vi "HOST_feedback+datatrig_AAoptAOD_9-11-23.vi"() -> ()   [LabVIEW 2020]
uses:
  <vilib>/rvi/interface/nirviMethod/nirviMethod.xnode
  <vilib>/rvi/errors/niLvFpgaMergeErrorWithErrorCode.vi
  <instrlib>/_niInstr/Streaming/v1/Host/niInstr Streaming v1 Host.lvlib
  <vilib>/rvi/interface/nirviReadWriteControl/nirviReadWriteControl.xnode
  <vilib>/rvi/interface/nirviCloseFPGA/nirviCloseFPGA.xnode
  <vilib>/rvi/interface/nirviOpenFPGA/nirviOpenFPGA.xnode
  <vilib>/rvi/interface/Simulation/niFpgaSimulationCallBeginRW.vi
  <vilib>/rvi/errors/niLvFpgaAdjustHostInterfaceError.vi
  NiFpgaLv.dll
  <vilib>/Utility/error.llb/Error Cluster From Error Code.vi
  <vilib>/Utility/file.llb/Write Delimited Spreadsheet (string).vi
  <instrlib>/_niInstr/Streaming/v1/Host/Public/Start Finite Stream.vi
  <instrlib>/_niInstr/Streaming/v1/Host/Public/Wait for Stream.vi
  <vilib>/FPGAPlugInAG/Dynamic/niLvFpga_ConfigureFifo_Dynamic.vi
  <vilib>/FPGAPlugInAG/Dynamic/niLvFpga_StartFifo_Dynamic.vi
  <vilib>/FPGAPlugInAG/Dynamic/niLvFpga_ReadFifo_Dynamic.vi
  <vilib>/FPGAPlugInAG/Dynamic/niLvFpga_WriteFifo_Dynamic.vi
  <vilib>/FPGAPlugInAG/Dynamic/niLvFpga_Close_Dynamic.vi
  FPGA Bitfiles/rfsignal_FPGATarget_feedbackarray+da_BHXJFx-D6v4.lvbitx
  <vilib>/measure/NI_MAPro.lvlib
  <instrlib>/_niInstr/Streaming/v1/Host/Public/Start Continuous Stream.vi
  <vilib>/measure/maspectr.llb/FFT Power Spectrum and PSD for N Chan.vi
  <vilib>/FPGAPlugInAG/PXIe-7972R/niLvFpga_Open_PXIe-7972R.vi
  <vilib>/rvi/interface/common/dynamic/niFpgaDynamicAddResources.vi
  <vilib>/userdefined/Silver/nirio_resource_slv.ctl
  Controls/Clock Select.ctl
  PID/Typedef/niFpgaPID_PIDGains.ctl
  PID/Typedef/niFpgaPID_OutputRange.ctl
  PID/Typedef/niFpgaPID_SetpointWeightings.ctl
  PID/Typedef/niFpgaPID_PIDActions.ctl
panel:
  in  "RF Power normalize":bool=TRUE
  in  "Save data":bool
  in  "File name":string="Z_3mbar_i"
  in  "Save Path Directory":path=path "D:/Lab Data/test"
  out "SUM PSD":cluster{"f0":dbl, "df":dbl, "magnitude":dbl[]}[](graph)
  out "SUM":waveform(dbl)[](graph)=[{"t0"=timestamp(0 s since 1904-01-01), "dt"=0.0002, "Y"=array[1000 elements]}, {"t0"=timestamp(0 s since 1904-01-01), "dt"=0.0002, "Y"=array[1000 elements]}, {"t0"=timestamp(0 s since 1904-01-01), "dt"=0.0002, "Y"=array[1000 elements]}, {"t0"=timestamp(0 s since 1904-01-01), "dt"=0.0002, "Y"=array[1000 elements]}]
  out "Y PSD":cluster{"f0":dbl, "df":dbl, "magnitude":dbl[]}[](graph)
  out "Y":waveform(dbl)[](graph)=[{"t0"=timestamp(0 s since 1904-01-01), "dt"=0.0002, "Y"=array[1000 elements]}, {"t0"=timestamp(0 s since 1904-01-01), "dt"=0.0002, "Y"=array[1000 elements]}, {"t0"=timestamp(0 s since 1904-01-01), "dt"=0.0002, "Y"=array[1000 elements]}, {"t0"=timestamp(0 s since 1904-01-01), "dt"=0.0002, "Y"=array[1000 elements]}]
  out "X PSD":cluster{"f0":dbl, "df":dbl, "magnitude":dbl[]}[](graph)
  out "X":waveform(dbl)[](graph)=[{"t0"=timestamp(0 s since 1904-01-01), "dt"=0.0002, "Y"=array[1000 elements]}, {"t0"=timestamp(0 s since 1904-01-01), "dt"=0.0002, "Y"=array[1000 elements]}, {"t0"=timestamp(0 s since 1904-01-01), "dt"=0.0002, "Y"=array[1000 elements]}, {"t0"=timestamp(0 s since 1904-01-01), "dt"=0.0002, "Y"=array[1000 elements]}]
  in  "Set Point Initialization":bool
  in  "Feedback scaling y":fxp<+,25,4>
  in  "Gains Y":T1[](array[typedef]) {"filter coefficient" min=0 max=1; "proportional gain" step=0.125}
  in  "Gains X":T1[](array[typedef]) {"filter coefficient" min=0 max=1; "proportional gain" step=0.125}
  in  "Data transfer method":bool
  in  "Downsample":u16=1
  in  "Signal Delay (us)":i32=5
  out "actions":T2
  out "error":sgl
  out "output":sgl
  out "error 2":sgl
  out "error 3":sgl
  out "output 3":sgl
  out "actions 3":T2
  out "output 2":sgl
  out "actions 2":T2
  in  "Gains Z":T1[](array[typedef]) {"filter coefficient" min=0 max=1; "proportional gain" step=0.125}
  in  "setpoint weighting 3":T3={"proportional weighting (1)"=1.0, "derivative weighting (0)"=0.0} {"derivative weighting (0)" min=0 max=1; "proportional weighting (1)" min=0 max=1}
  in  "output range 3":T4={"output high (Inf)"=inf, "output low (-Inf)"=-inf}
  in  "Z reset? (F)":bool
  in  "setpoint weighting 2":T3={"proportional weighting (1)"=1.0, "derivative weighting (0)"=0.0} {"derivative weighting (0)" min=0 max=1; "proportional weighting (1)" min=0 max=1}
  in  "output range 2":T4={"output high (Inf)"=inf, "output low (-Inf)"=-inf}
  in  "Y reset? (F)":bool
  in  "Feedback scaling z":fxp<+,32,4>
  in  "Feedback scaling x":fxp<+,25,4>
  in  "Apply feedback":bool
  in  "Data Trigger Level (V)":dbl
  in  "Record Size":u32=1024
  out "AI":waveform(dbl)[](graph)
  in  "Data Trigger When":enum8{"Trigger Above", "Trigger Below"}(ring)
  in  "Trigger Type":enum8{"Immediate", "Data Trigger", "TRIG input"}(ring)
  in  "Direction switch":bool
  in  "Step gain values":dbl
  in  "?":bool
  in  "% of max CH 1":dbl=85.0
  in  "% of max CH 0":dbl=90.0
  in  "setpoint weighting":T3={"proportional weighting (1)"=1.0, "derivative weighting (0)"=0.0} {"derivative weighting (0)" min=0 max=1; "proportional weighting (1)" min=0 max=1}
  in  "output range":T4={"output high (Inf)"=inf, "output low (-Inf)"=-inf}
  in  "X reset? (F)":bool
  in  "write time ch0":bool
  in  "Record time for power sweep CH0":bool
  in  "Record time for power sweep CH1":bool
  in  "write time ch1":bool
  in  "save path for power calibration (dialog if empty)":path
  out "time check":u16=16
  in  "Cycles per step":u16=30
  in  "Gain Scan Endpoint (CH1)":dbl[](array[numeric])=[100.0, 100.0, 100.0, 100.0, 100.0, 100.0, 100.0, 100.0, 100.0, 100.0, 100.0, 100.0, 100.0, 100.0, 100.0, 100.0, 100.0, 100.0, 100.0, 100.0, 100.0, 100.0, 100.0, 100.0, 100.0, 100.0, 100.0, 100.0, 100.0, 100.0, 100.0, 100.0, 100.0, 100.0, 100.0, 100.0]
  in  "Gain Scan Endpoint (CH0)":dbl[](array[numeric])=[100.0, 100.0, 100.0, 100.0, 100.0, 100.0, 100.0, 100.0, 100.0, 100.0, 100.0, 100.0, 100.0, 100.0, 100.0, 100.0, 100.0, 100.0, 100.0, 100.0, 100.0, 100.0, 100.0, 100.0, 100.0, 100.0, 100.0, 100.0, 100.0, 100.0, 100.0, 100.0, 100.0, 100.0, 100.0, 100.0]
  in  "Scan End Setpoint (CH1)":dbl[](array[numeric])=[23.0, 24.0, 25.0, 26.0, 27.0, 28.0, 23.0, 24.0, 25.0, 26.0, 27.0, 28.0, 23.0, 24.0, 25.0, 26.0, 27.0, 28.0, 23.0, 24.0, 25.0, 26.0, 27.0, 28.0, 23.0, 24.0, 25.0, 26.0, 27.0, 28.0, 23.0, 24.0, 25.0, 26.0, 27.0, 28.0] format="%#_10f"
  in  "Scan CH1":bool
  in  "Scan CH0":bool
  in  "Fq Scan Endpoint (CH0)":dbl[](array[numeric])=[23.0, 23.0, 23.0, 23.0, 23.0, 23.0, 24.0, 24.0, 24.0, 24.0, 24.0, 24.0, 25.0, 25.0, 25.0, 25.0, 25.0, 25.0, 26.0, 26.0, 26.0, 26.0, 26.0, 26.0, 27.0, 27.0, 27.0, 27.0, 27.0, 27.0, 28.0, 28.0, 28.0, 28.0, 28.0, 28.0] format="%#_10f"
  in  "Gain Scan Step Size % (CH1)":dbl=1.0
  in  "Gain Scan Step Size % (CH0)":dbl=1.0
  in  "Fq Scan Step Size MHz (CH1)":dbl=0.1
  in  "Fq Scan Step Size MHz (CH0)":dbl=0.1
  in  "Input pass through\nmode":enum16{"Wire", "Accum-edge"}(ring)=enum."Accum-edge"
  in  "# of beams":u8=36
  in  "Wave Reader CH 1 (MHz)":dbl[](array[numeric])=[23.0, 24.0, 25.0, 26.0, 27.0, 28.0, 23.0, 24.0, 25.0, 26.0, 27.0, 28.0, 23.0, 24.0, 25.0, 26.0, 27.0, 28.0, 23.0, 24.0, 25.0, 26.0, 27.0, 28.0, 23.0, 24.0, 25.0, 26.0, 27.0, 28.0, 23.0, 24.0, 25.0, 26.0, 27.0, 28.0] format="%#_15f"
  in  "Gain CH 1 (%)":dbl[](array[numeric])=[100.0, 100.0, 100.0, 100.0, 100.0, 100.0, 100.0, 100.0, 100.0, 100.0, 100.0, 100.0, 100.0, 100.0, 100.0, 100.0, 100.0, 100.0, 100.0, 100.0, 100.0, 100.0, 100.0, 100.0, 100.0, 100.0, 100.0, 100.0, 100.0, 100.0, 100.0, 100.0, 100.0, 100.0, 100.0, 100.0]
  in  "Remove transition edges":i32=5
  in  "Time per beam in us":i32=20
  in  "stop":bool
  in  "Gain CH 0 (%)":dbl[](array[numeric])=[100.0, 100.0, 100.0, 100.0, 100.0, 100.0, 100.0, 100.0, 100.0, 100.0, 100.0, 100.0, 100.0, 100.0, 100.0, 100.0, 100.0, 100.0, 100.0, 100.0, 100.0, 100.0, 100.0, 100.0, 100.0, 100.0, 100.0, 100.0, 100.0, 100.0, 100.0, 100.0, 100.0, 100.0, 100.0, 100.0]
  in  "Wave Reader CH 0 (MHz)":dbl[](array[numeric])=[23.0, 23.0, 23.0, 23.0, 23.0, 23.0, 24.0, 24.0, 24.0, 24.0, 24.0, 24.0, 25.0, 25.0, 25.0, 25.0, 25.0, 25.0, 26.0, 26.0, 26.0, 26.0, 26.0, 26.0, 27.0, 27.0, 27.0, 27.0, 27.0, 27.0, 28.0, 28.0, 28.0, 28.0, 28.0, 28.0] format="%#_13f"
  in  "Magnitude Initialization Vpp":dbl[](array[numeric])=[1.0, 1.0] format="%0.2p"
  in  "Frequencies (Hz)":dbl[](array[numeric])=[10000.0, 10000.0] format="%5.0p"
  in  "Signal Type":T5(ring)
  in  "Sampling Info":cluster{"Fs":dbl, "#s":dbl}={"Fs"=163840000.0, "#s"=65536.0} {"Fs" format="%#_5p"}
  out "Error Out":errorcluster
  in  "Update Waveform":bool
  in  "Clock Select":T6 items=["Internal Clock", "Internal Clock w/ Ref via CLK/REF IN", "Internal Clock w/ Ref via Sync Clock", "External Clock via CLK/REF IN"]
  in  "Rate of External Sample Clock (MHz)":u16=100 min=60 max=100 step=1
  in  "RIO Resource":T7="RIO0"
  # "Timeshare sampling doesn't work for 1 beam"
  # "General Feedback Settings"
  # "Time cycle loop processing"
  # "up to 65535"
  # "Don't change"
  # "Waveform Initialization"
  # "Controls the Output of the FPGA\nEach row corresponds to one beam created by the AOD\nCH 0 is Output 0 on the FPGA card and controls the () direction on the AOD; CH 1 is Output 1 on the FPGA card and controls the () direction on the AOD\n\nThe  set frequency is the output of the FPGA, this is then mixed with a 50MHz LO to be in the AOD's bandwidth of 75 +- 15MHz\n\nThe gain is the percentage of the 1Vpp initialized voltage to output. It is in percentage and goes from 0 - 100\n\nIt will play the first n rows of tones, \nwhere n is the \"# of beams\" value."
  # "DO NOT CHANGE"
  # "These allow you to smoothly ramp between frequencies or gain settings for each individual beam.\nThe channels scan independently, but it will simultaneously ramp every fq/gain in the channel to their desired point.\nThey should update to match the main control setting when scanning is not enabled."
  # "X Feedback"
  # "Use scaling factor around 0.003 \n(scales a 1 Vpp signal to 29 um displacement range)"
  # "Do not change these values while waiting for scan"
  # "Main control for the tones played on FPGA analog out 0\nSets the base, static frequency to play"
  # "Main control for the tones played on FPGA analog out 1\nSets the base, static frequency to play"
  # "Ch 0 Output Waveforms"
  # "Ch 1 Output Waveforms"
  # "Y Feedback"
  # "Ch0"
  # "Use scaling factor around 0.003 \n(scales a 1 Vpp signal to 29 um displacement range)"
  # "Ch1"
  # "Makes sure the RF power into the\nAOD is flattened to 1.7W across the\nbandwidth\nDO NOT TURN OFF UNLESS YOU\nARE CALIBRATING POWERS!"
  # "Z Feedback"
  # "Use scaling factor around 6.62E-6 \n(scales a 1 Vpp signal to 15% gain range)"
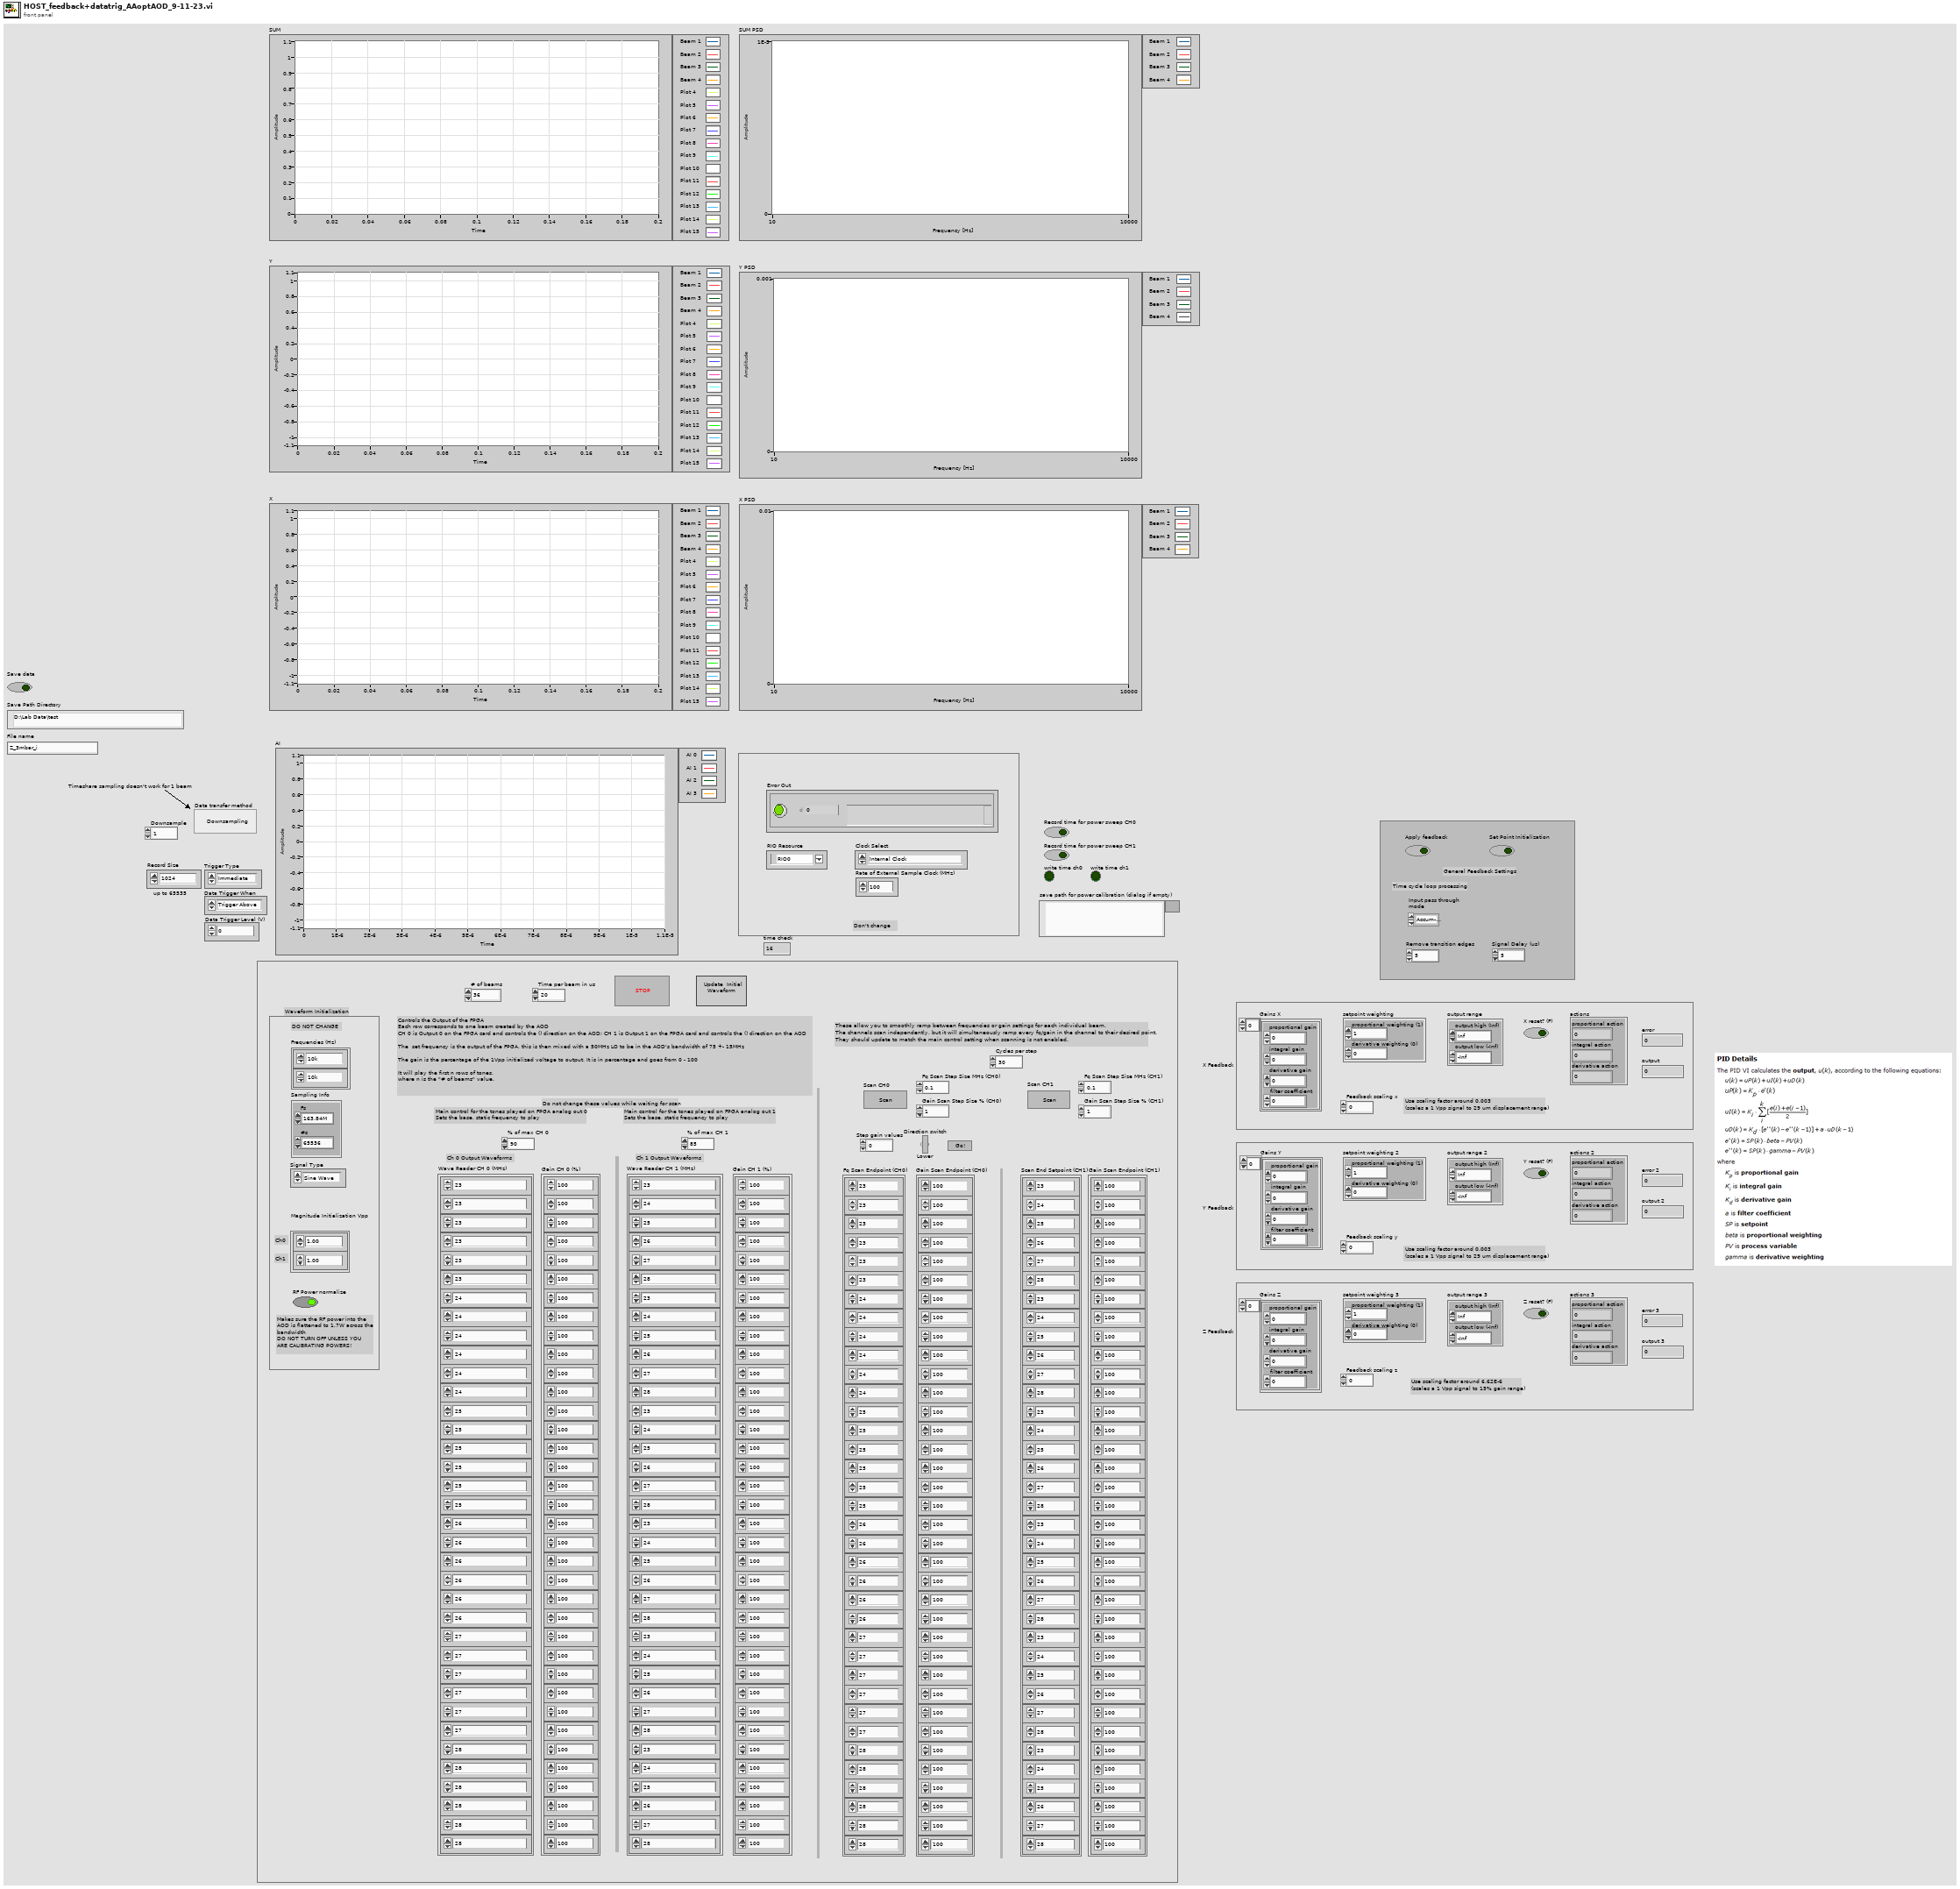
[diagram p1: front panel]
types:
  T1 = typedef "niFpgaPID_PIDGains.ctl" = cluster{"proportional gain":sgl, "integral gain":sgl, "derivative gain":sgl, "filter coefficient":sgl}
  T2 = typedef "niFpgaPID_PIDActions.ctl" = cluster{"proportional action":sgl, "integral action":sgl, "derivative action":sgl}
  T3 = typedef "niFpgaPID_SetpointWeightings.ctl" = cluster{"proportional weighting (1)":sgl, "derivative weighting (0)":sgl}
  T4 = typedef "niFpgaPID_OutputRange.ctl" = cluster{"output high (Inf)":sgl, "output low (-Inf)":sgl}
  T5 = enum16{"Sine Wave", "Triangle Wave", "Square Wave", "Sawtooth Wave"}
  T6 = typedef "Clock Select.ctl" = u16
  T7 = typedef "nirio_resource_slv.ctl" = tag
  T8 = cluster{"proportional action":sgl, "integral action":sgl, "derivative action":sgl}
  T9 = cluster{"level":i16, "trigger when":enum8{"Trigger Above", "Trigger Below"}}
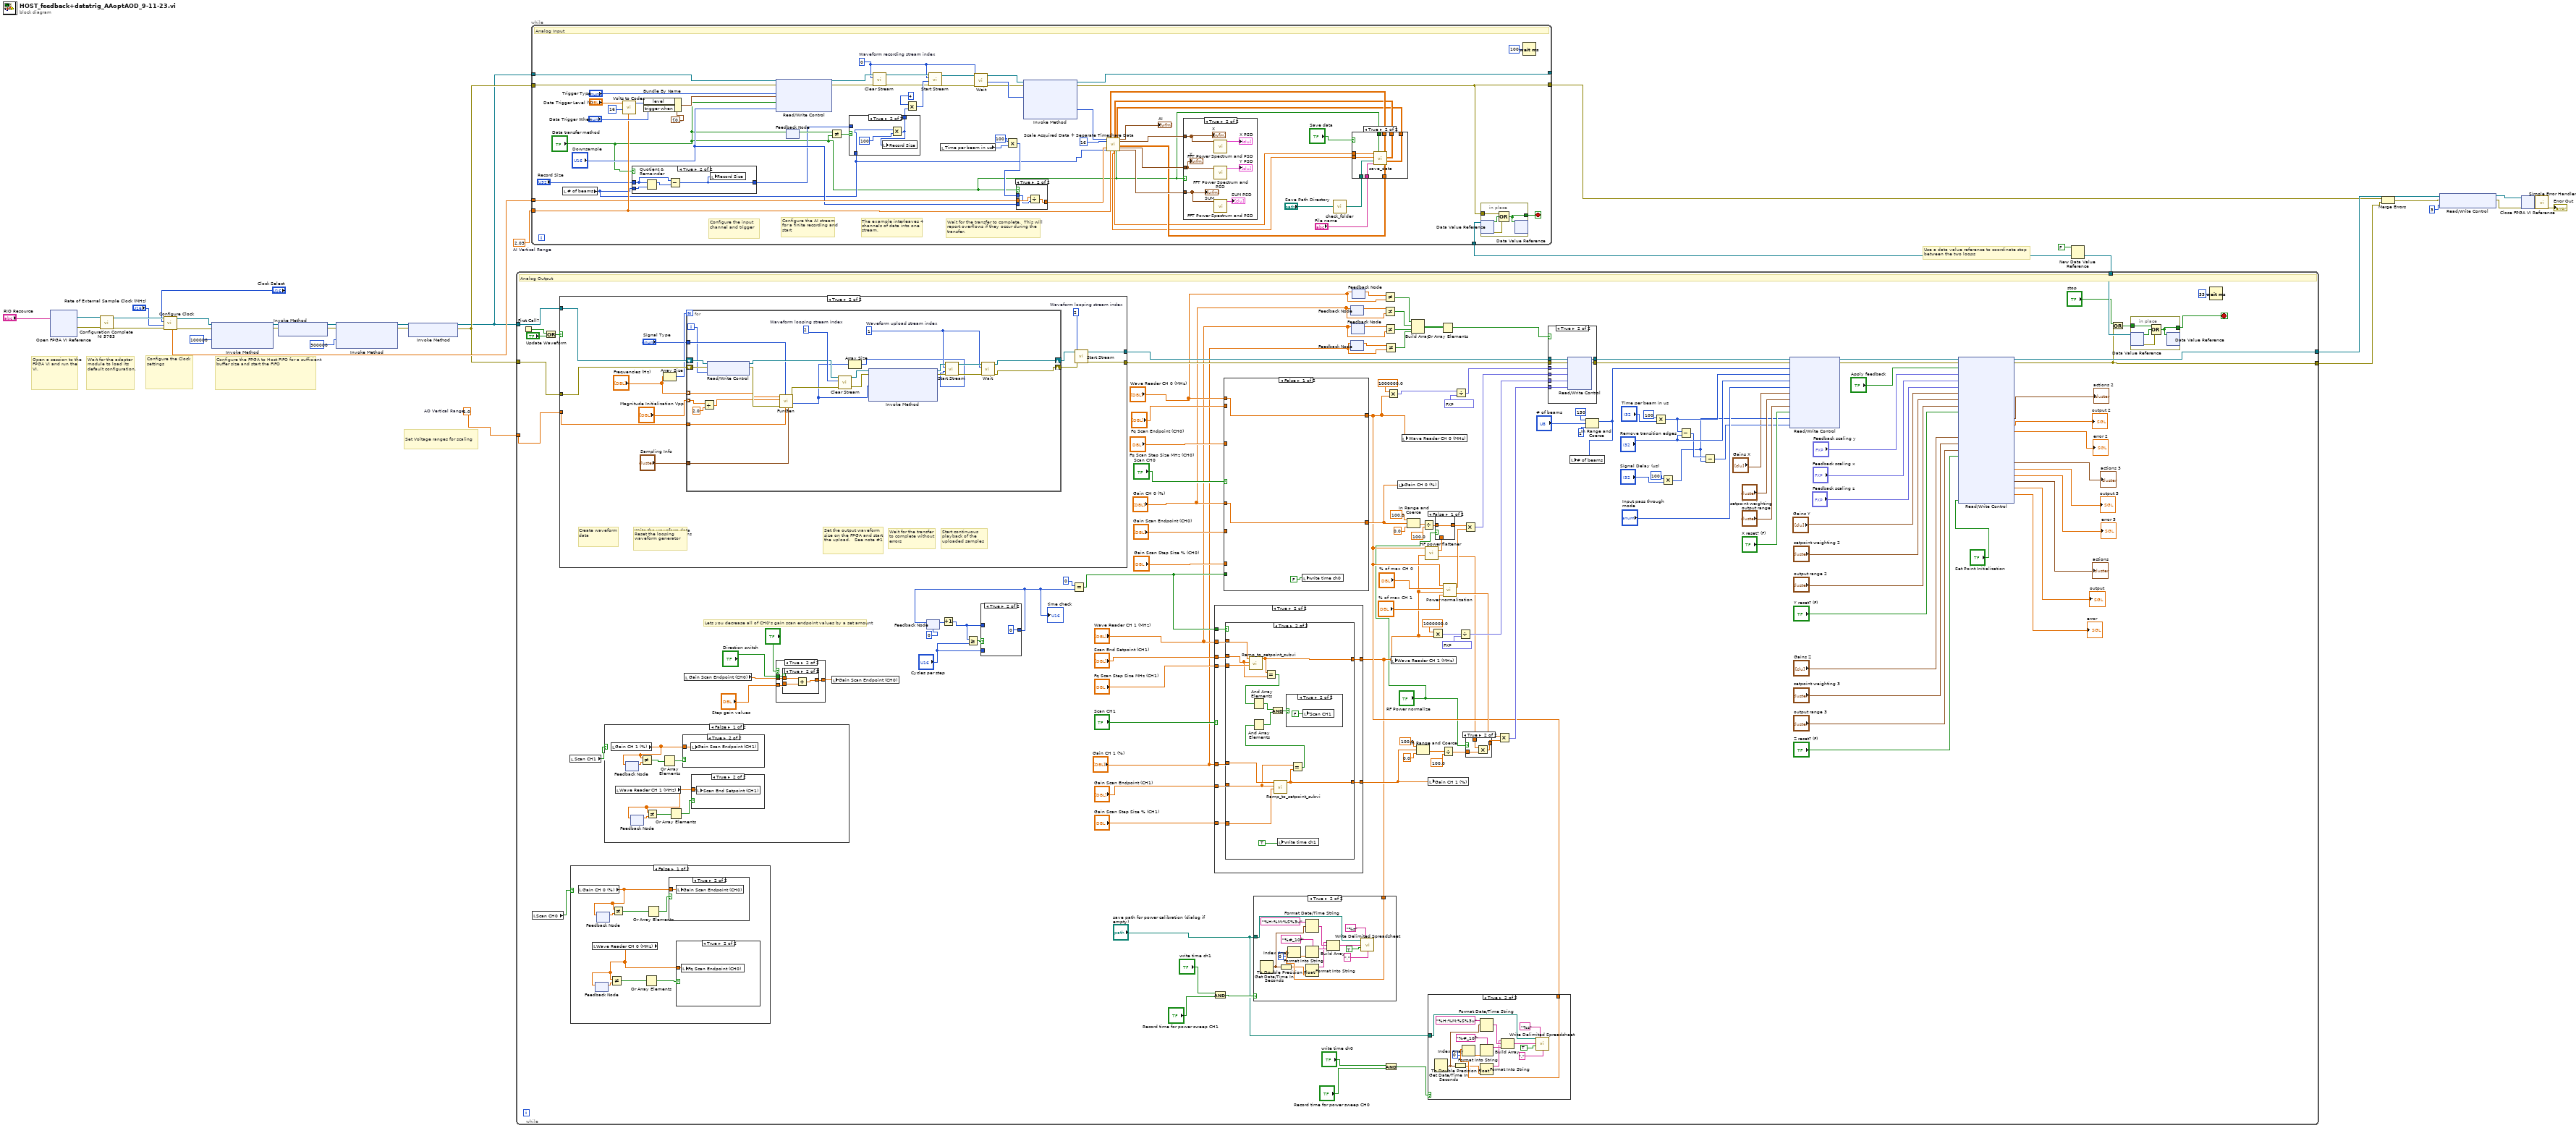
[diagram p0: block diagram]
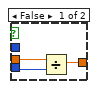
[diagram p6: hidden frame]
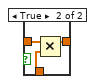
[diagram p8: hidden frame]
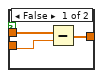
[diagram p11: hidden frame]
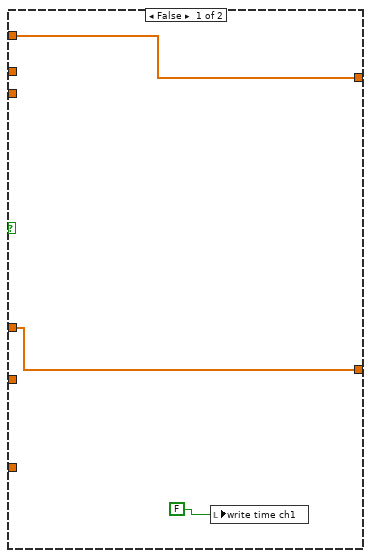
[diagram p14: hidden frame]
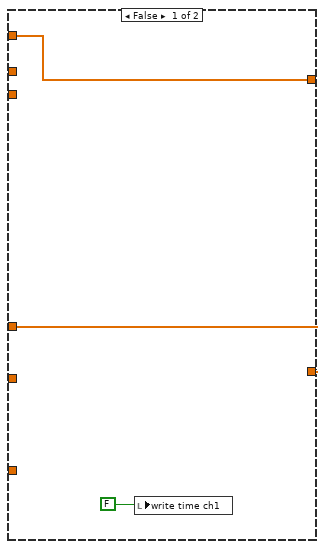
[diagram p15: hidden frame]
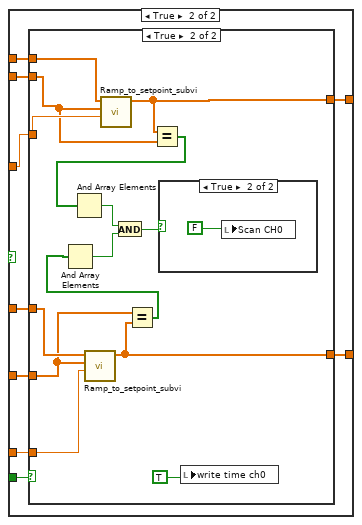
[diagram p17: hidden frame]
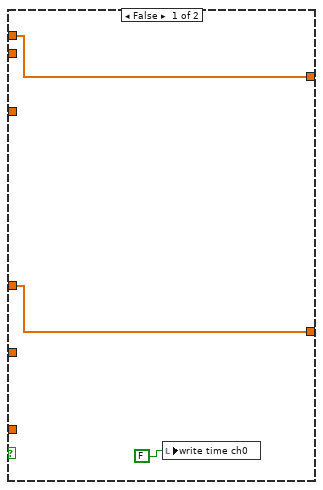
[diagram p18: hidden frame]
diagram:
  w13 = 2.03  # AI Vertical Range
  w21 = 1.0  # AO Vertical Range
  # "Use a data value reference to coordinate stop between the two loops"
  # "Set Voltage ranges for scaling"
  # "Configure the Clock settings"
  # "Configure the FPGA to Host FIFO for a sufficient buffer size and start the FIFO"
  # "Wait for the adapter module to load its default configuration."
  # "Open a session to the FPGA VI and run the VI."
  n1 = xnode "Open FPGA VI Reference"("resource name"="RIO Resource") -> ("FPGA VI Reference Out"=w19:refnum<k20>, "error out"=w18:errorcluster)  [unwired: 1 in]
  n2 = call "Configuration Complete NI 5783.vi"("error in"=w18, "FPGA VI Reference In"=w19) -> ("error out"=w29:errorcluster, "FPGA VI Reference Out"=w30:refnum<k20>)  [unwired: 7 in, 1 out]
  n3 = call "Configure Clock.vi"("error in (no error)"=w29, "Rate of External Sample Clock (MHz)"="Rate of External Sample Clock (MHz)", "Clock Select"="Clock Select", "FPGA VI Reference In"=w30) -> ("error out"=w27:errorcluster, "FPGA VI Reference Out"=w28:refnum<k20>, "Sampling Rate"=w12:dbl)  [unwired: 3 in, 2 out]
  n4 = xnode "Invoke Method"("FPGA VI Reference In"=w28, "error in"=w27, "Requested Depth"=u32 100000) -> ("FPGA VI Reference Out"=w33:refnum<k20>, "error out"=w32:errorcluster)  [unwired: 1 out]
  n5 = xnode "Invoke Method"("FPGA VI Reference In"=w33, "error in"=w32) -> ("FPGA VI Reference Out"=w5:refnum<k20>, "error out"=w8:errorcluster)
  n6 = xnode "Invoke Method"("FPGA VI Reference In"=w5, "error in"=w8, "Requested Depth"=u32 300000) -> ("FPGA VI Reference Out"=w4:refnum<k20>, "error out"=w7:errorcluster)  [unwired: 1 out]
  n7 = xnode "Invoke Method"("FPGA VI Reference In"=w4, "error in"=w7) -> ("FPGA VI Reference Out"=w3:refnum<k20>, "error out"=w6:errorcluster)
  n8 = New Data Value Reference(data value=FALSE ("Stopped")) -> (data value reference=w1:refnum<data-value>)  [unwired: 1 in, 1 out]
  n9 = while {
    tunnel: w6 -> [w165]
    tunnel: w3 -> [w171]
    tunnel: [w91] -> w17
    tunnel: w1 -> [w166]
    tunnel: w21 -> [w164]
    tunnel: [w89] -> w9
    stop <- w96 stop-if-true
    # "Lets you decrease all of CH0's gain scan endpoint values by a set amount"
    # "Analog Output"
    n10 = First Call?() -> (First Call?: T/F=w167:bool)
    n11 = local read "Scan CH0"() -> (w134:bool)
    n12 = Or(x=w167, y="Update Waveform") -> (x .or. y?=w168:bool)
    n13 = case shown="True" w168 {
      tunnel: [w318 w331] -> w163
      tunnel: [w317 w330] -> w162
      tunnel: w171 -> [w318 w328]
      tunnel: w165 -> [w317 w327]
      tunnel: w164 -> [_ w329]
      frame False {
      }
      frame True {
        w326 = 2  # Waveform looping stream index
        # "Loop over the waveforms to combine"
        # "Reset the looping waveform generator"
        # "Start continuous playback of the uploaded samples"
        # "Wait for the transfer to complete without errors"
        # "Set the output waveform size on the FPGA and start the upload.   See note #1"
        # "Write the waveform data to the FPGA for generation"
        # "Create waveform data"
        n14 = Array Size(array="Frequencies (Hz)") -> (size(s)=w321:i32)
        n15 = for {
          N: w321 -> [_]
          tunnel: w329 -> [w346]
          shift-right: [w340] -> w325
          shift-left: w328 -> [w345]
          shift-right: [w339] -> w324
          shift-left: w327 -> [w343]
          tunnel: "Frequencies (Hz)" -> [w338] mode=indexing
          tunnel: "Magnitude Initialization Vpp" -> [w334] mode=indexing
          tunnel: "Sampling Info" -> [w337]
          tunnel: "Signal Type" -> [w336]
          i -> [w335]
          w347 = 2  # Waveform looping stream index
          w352 = 1  # Waveform upload stream index
          n16 = Divide(x=w334, y=2.0) -> (x/y=w333:dbl)
          n17 = xnode "Read/Write Control"("FPGA VI Reference In"=w345, "error in"=w343, "Upload selector"=w335) -> ("FPGA VI Reference Out"=w344:refnum<k20>, "error out"=w342:errorcluster)
          n18 = call "FunGen.vi"("sampling info"=w337, "range (Vpp)"=w346, "signal type"=w336, "error in (no error)"=w342, "amplitude"=w333, "frequency"=w338) -> ("error out"=w348:errorcluster, "Waveform Data"=w341:i16[])  [unwired: 2 in, 2 out]
          n19 = call <instrlib>:"Clear Stream.vi"("error in (no error)"=w348, "stream index"=w347, "refnum in"=w344) -> ("error out"=w350:errorcluster, "refnum out"=w351:refnum<k20>)  [unwired: 7 in]
          n20 = Array Size(array=w341) -> (size(s)=w349:i32)
          n21 = xnode "Invoke Method"("FPGA VI Reference In"=w351, "error in"=w350, "Data"=w341) -> ("FPGA VI Reference Out"=w356:refnum<k20>, "error out"=w355:errorcluster)  [unwired: 1 in, 1 out]
          n22 = call-poly <instrlib>:"Start Stream.vi"("error in (no error)"=w355, "num samples"=w349, "stream index"=w352, "refnum in"=w356) -> ("error out"=w353:errorcluster, "refnum out"=w354:refnum<k20>)  [unwired: 6 in]
          n23 = call-poly <instrlib>:"Wait.vi"("error in (no error)"=w353, "stream index"=w352, "refnum in"=w354) -> ("error out"=w339:errorcluster, "refnum out"=w340:refnum<k20>)  [unwired: 5 in, 2 out]
        }
        n24 = call-poly <instrlib>:"Start Stream.vi"("error in (no error)"=w324, "stream index"=w326, "refnum in"=w325) -> ("error out"=w330:errorcluster, "refnum out"=w331:refnum<k20>)  [unwired: 7 in]
      }
    }
    n25 = local read "Scan CH1"() -> (w135:bool)
    n26 = case shown="False" w134 {
      frame False {
        n27 = local read "Gain CH 0 (%)"() -> (w293:dbl[])
        n28 = local read "Wave Reader CH 0 (MHz)"() -> (w300:dbl[])
        n29 = feedback-in #1(w300) -> ()
        n30 = feedback #1() -> (w299:dbl[])  [unwired: 1 in]
        n31 = feedback #2() -> (w296:dbl[])  [unwired: 1 in]
        n32 = feedback-in #2(w293) -> ()
        n33 = Not Equal?(x=w300, y=w299) -> (x != y?=w298:bool[])
        n34 = Not Equal?(x=w293, y=w296) -> (x != y?=w295:bool[])
        n35 = Or Array Elements(Boolean array=w298) -> (logical OR=w297:bool)
        n36 = Or Array Elements(Boolean array=w295) -> (logical OR=w294:bool)
        n37 = case shown="True" w294 {
          tunnel: w293 -> [_ w301]
          frame False {
          }
          frame True {
            n38 = local write "Gain Scan Endpoint (CH0)"(w301) -> ()
          }
        }
        n39 = case shown="True" w297 {
          tunnel: w300 -> [_ w302]
          frame False {
          }
          frame True {
            n40 = local write "Fq Scan Endpoint (CH0)"(w302) -> ()
          }
        }
      }
      frame True {
      }
    }
    n41 = case shown="False" w135 {
      frame False {
        n42 = local read "Gain CH 1 (%)"() -> (w303:dbl[])
        n43 = local read "Wave Reader CH 1 (MHz)"() -> (w307:dbl[])
        n44 = feedback #3() -> (w306:dbl[])  [unwired: 1 in]
        n45 = feedback-in #3(w303) -> ()
        n46 = feedback #4() -> (w310:dbl[])  [unwired: 1 in]
        n47 = feedback-in #4(w307) -> ()
        n48 = Not Equal?(x=w303, y=w306) -> (x != y?=w305:bool[])
        n49 = Not Equal?(x=w307, y=w310) -> (x != y?=w309:bool[])
        n50 = Or Array Elements(Boolean array=w305) -> (logical OR=w304:bool)
        n51 = Or Array Elements(Boolean array=w309) -> (logical OR=w308:bool)
        n52 = case shown="True" w304 {
          tunnel: w303 -> [_ w311]
          frame False {
          }
          frame True {
            n53 = local write "Gain Scan Endpoint (CH1)"(w311) -> ()
          }
        }
        n54 = case shown="True" w308 {
          tunnel: w307 -> [_ w312]
          frame False {
          }
          frame True {
            n55 = local write "Scan End Setpoint (CH1)"(w312) -> ()
          }
        }
      }
      frame True {
      }
    }
    n56 = local read "Gain Scan Endpoint (CH0)"() -> (w98:dbl[])
    n57 = case shown="True" "?" {
      tunnel: w98 -> [w190 w193]
      tunnel: [w190 w194] -> w99
      tunnel: "Step gain values" -> [_ w192]
      tunnel: "Direction switch" -> [_ w191]
      frame False {
      }
      frame True {
        n58 = case shown="True" w191 {
          tunnel: [w197 w199] -> w194
          tunnel: w193 -> [w196 w198]
          tunnel: w192 -> [w195 w200]
          frame False {
            n59 = Subtract(x=w196, y=w195) -> (x-y=w197:dbl[])
          }
          frame True {
            n60 = Add(x=w198, y=w200) -> (x+y=w199:dbl[])
          }
        }
      }
    }
    n61 = local write "Gain Scan Endpoint (CH0)"(w99) -> ()
    n62 = feedback #5(u16 0) -> (w130:u16)
    n63 = Increment(x=w130) -> (x+1=w128:u16)
    n64 = Greater Or Equal?(x=w128, y="Cycles per step") -> (x >= y?=w129:bool)
    n65 = case shown="True" w129 {
      tunnel: w128 -> [w291 _]
      tunnel: "Cycles per step" -> [_ _]
      tunnel: [w291 u16 0] -> w123
      frame False {
      }
      frame True {
      }
    }
    "time check" <- w123
    n66 = feedback-in #5(w123) -> ()
    n67 = Equal?(x=u16 0, y=w123) -> (x = y?=w124:bool)
    n68 = And(x="write time ch1", y="Record time for power sweep CH1") -> (x .and. y?=w122:bool)
    n69 = case shown="True" "Scan CH1" {
      tunnel: "Fq Scan Step Size MHz (CH1)" -> [_ w242]
      tunnel: [w233 w241] -> w56
      tunnel: "Wave Reader CH 1 (MHz)" -> [w233 w240]
      tunnel: "Scan End Setpoint (CH1)" -> [_ w239]
      tunnel: "Gain Scan Step Size % (CH1)" -> [_ w238]
      tunnel: "Gain CH 1 (%)" -> [w232 w237]
      tunnel: "Gain Scan Endpoint (CH1)" -> [_ w236]
      tunnel: [w232 w235] -> w136
      tunnel: w124 -> [_ w234]
      frame False {
        n70 = local write "write time ch1"(FALSE) -> ()
      }
      frame True {
        n71 = case shown="True" w234 {
          tunnel: w240 -> [w245 w259]
          tunnel: w239 -> [_ w257]
          tunnel: w242 -> [_ w258]
          tunnel: [w245 w256] -> w241
          tunnel: w237 -> [w244 w254]
          tunnel: w236 -> [_ w253]
          tunnel: w238 -> [_ w252]
          tunnel: [w244 w247] -> w235
          frame False {
            n72 = local write "write time ch1"(FALSE) -> ()
          }
          frame True {
            n73 = call "Ramp_to_setpoint_subvi.vi"("Numeric"=w258, "Scan to Fq (CH0)"=w257, "Wave Reader CH 0 (Y)"=w259) -> ("Array"=w256:dbl[])  [unwired: 8 in]
            n74 = Equal?(x=w256, y=w257) -> (x = y?=w255:bool[])
            n75 = And Array Elements(Boolean array=w255) -> (logical AND=w249:bool)
            n76 = call "Ramp_to_setpoint_subvi.vi"("Numeric"=w252, "Scan to Fq (CH0)"=w253, "Wave Reader CH 0 (Y)"=w254) -> ("Array"=w247:dbl[])  [unwired: 8 in]
            n77 = local write "write time ch1"(TRUE) -> ()
            n78 = Equal?(x=w253, y=w247) -> (x = y?=w248:bool[])
            n79 = And Array Elements(Boolean array=w248) -> (logical AND=w250:bool)
            n80 = And(x=w249, y=w250) -> (x .and. y?=w251:bool)
            n81 = case shown="True" w251 {
              frame False {
              }
              frame True {
                n82 = local write "Scan CH1"(FALSE) -> ()
              }
            }
          }
        }
      }
    }
    n83 = case shown="False" "Scan CH0" {
      tunnel: "Fq Scan Step Size MHz (CH0)" -> [_ w272]
      tunnel: "Wave Reader CH 0 (MHz)" -> [w263 w271]
      tunnel: "Fq Scan Endpoint (CH0)" -> [_ w270]
      tunnel: [w263 w269] -> w59
      tunnel: "Gain CH 0 (%)" -> [w262 w268]
      tunnel: "Gain Scan Endpoint (CH0)" -> [_ w267]
      tunnel: [w262 w266] -> w143
      tunnel: "Gain Scan Step Size % (CH0)" -> [_ w265]
      tunnel: w124 -> [_ w264]
      frame False {
        n84 = local write "write time ch0"(FALSE) -> ()
      }
      frame True {
        n85 = case shown="True" w264 {
          tunnel: w271 -> [w275 w289]
          tunnel: w270 -> [_ w287]
          tunnel: w272 -> [_ w288]
          tunnel: [w275 w286] -> w269
          tunnel: w268 -> [w274 w284]
          tunnel: w267 -> [_ w281]
          tunnel: w265 -> [_ w283]
          tunnel: [w274 w282] -> w266
          frame False {
            n86 = local write "write time ch0"(FALSE) -> ()
          }
          frame True {
            n87 = call "Ramp_to_setpoint_subvi.vi"("Numeric"=w283, "Scan to Fq (CH0)"=w281, "Wave Reader CH 0 (Y)"=w284) -> ("Array"=w282:dbl[])  [unwired: 8 in]
            n88 = call "Ramp_to_setpoint_subvi.vi"("Numeric"=w288, "Scan to Fq (CH0)"=w287, "Wave Reader CH 0 (Y)"=w289) -> ("Array"=w286:dbl[])  [unwired: 8 in]
            n89 = Equal?(x=w281, y=w282) -> (x = y?=w280:bool[])
            n90 = And Array Elements(Boolean array=w280) -> (logical AND=w277:bool)
            n91 = Equal?(x=w286, y=w287) -> (x = y?=w285:bool[])
            n92 = And Array Elements(Boolean array=w285) -> (logical AND=w278:bool)
            n93 = And(x=w278, y=w277) -> (x .and. y?=w279:bool)
            n94 = case shown="True" w279 {
              frame False {
              }
              frame True {
                n95 = local write "Scan CH0"(FALSE) -> ()
              }
            }
            n96 = local write "write time ch0"(TRUE) -> ()
          }
        }
      }
    }
    n97 = case shown="True" w122 {
      tunnel: w56 -> [_ w223]
      tunnel: "save path for power calibration (dialog if empty)" -> [_ w216]
      frame False {
      }
      frame True {
        n98 = Get Date/Time In Seconds() -> (seconds since 1Jan1904=w219:timestamp)
        n99 = To Double Precision Float(number=w219) -> (double precision float=w218:dbl)
        n100 = Index Array(array=w223, index=0) -> (element=w221:dbl)
        n101 = Format Date/Time String(time format string (%c)="%H:%M:%S%3u", seconds (now)=w219) -> (date/time string=w226:string)  [unwired: 1 in]
        n102 = Format Into String(format string="%#_10f", w221) -> (resulting string=w225:string)  [unwired: 2 in, 1 out]
        n103 = Format Into String(w218) -> (resulting string=w217:string)  [unwired: 3 in, 1 out]
        n104 = Build Array(w217, w226, w225) -> (w220:string[])
        n105 = call-poly <vilib>:"Write Delimited Spreadsheet.vi"("file path (dialog if empty)"=w216, "format (%s)"="%s" ("format (%.3f)"), "1D data"=w220, "append to file? (new file:F)"=TRUE, "delimiter (\\t)"="," ("delimiter (\\t)")) -> ()  [unwired: 9 in, 2 out]
      }
    }
    n106 = feedback-in #6("Gain CH 0 (%)") -> ()
    n107 = feedback #6() -> (w50:dbl[])  [unwired: 1 in]
    n108 = feedback #7() -> (w46:dbl[])  [unwired: 1 in]
    n109 = feedback-in #7("Gain CH 1 (%)") -> ()
    n110 = feedback #8() -> (w48:dbl[])  [unwired: 1 in]
    n111 = feedback-in #8("Wave Reader CH 1 (MHz)") -> ()
    n112 = feedback #9() -> (w51:dbl[])  [unwired: 1 in]
    n113 = feedback-in #9("Wave Reader CH 0 (MHz)") -> ()
    n114 = Not Equal?(x=w51, y="Wave Reader CH 0 (MHz)") -> (x != y?=w44:bool[])
    n115 = Not Equal?(x=w50, y="Gain CH 0 (%)") -> (x != y?=w43:bool[])
    n116 = Not Equal?(x=w48, y="Wave Reader CH 1 (MHz)") -> (x != y?=w42:bool[])
    n117 = Not Equal?(x=w46, y="Gain CH 1 (%)") -> (x != y?=w41:bool[])
    n118 = And(x="write time ch0", y="Record time for power sweep CH0") -> (x .and. y?=w118:bool)
    n119 = Multiply(x=1000000.0, y=w59) -> (x*y=w152:fxp<+/-,64,32>[])
    n120 = local write "Wave Reader CH 1 (MHz)"(w56) -> ()
    n121 = local write "Gain CH 0 (%)"(w143) -> ()
    n122 = local write "Wave Reader CH 0 (MHz)"(w59) -> ()
    n123 = In Range and Coerce(upper limit=100.0, x=w143, lower limit=0.0) -> (coerced(x)=w146:dbl[])  [unwired: 1 out]
    n124 = Build Array(w44, w43, w42, w41) -> (w40:bool[][])
    n125 = In Range and Coerce(upper limit=100.0, x=w136, lower limit=0.0) -> (coerced(x)=w141:dbl[])  [unwired: 1 out]
    n126 = Divide(x=w146, y=100.0) -> (x/y=w109:dbl[])
    n127 = call "HF power flattener.vi"("CH 1 frequency"=w56, "CH 0 frequency"=w59) -> ("Normalized CH1"=w53:dbl[], "Normalized CH 0"=w57:dbl[])  [unwired: 2 in]
    n128 = local write "Gain CH 1 (%)"(w136) -> ()
    n129 = case shown="True" w118 {
      tunnel: w59 -> [_ w208]
      tunnel: "save path for power calibration (dialog if empty)" -> [_ w201]
      frame False {
      }
      frame True {
        n130 = Get Date/Time In Seconds() -> (seconds since 1Jan1904=w204:timestamp)
        n131 = To Double Precision Float(number=w204) -> (double precision float=w203:dbl)
        n132 = Index Array(array=w208, index=0) -> (element=w206:dbl)
        n133 = Format Date/Time String(time format string (%c)="%H:%M:%S%3u", seconds (now)=w204) -> (date/time string=w211:string)  [unwired: 1 in]
        n134 = Format Into String(format string="%#_10f", w206) -> (resulting string=w210:string)  [unwired: 2 in, 1 out]
        n135 = Format Into String(w203) -> (resulting string=w202:string)  [unwired: 3 in, 1 out]
        n136 = Build Array(w202, w211, w210) -> (w205:string[])
        n137 = call-poly <vilib>:"Write Delimited Spreadsheet.vi"("file path (dialog if empty)"=w201, "format (%s)"="%s" ("format (%.3f)"), "1D data"=w205, "append to file? (new file:F)"=TRUE, "delimiter (\\t)"="," ("delimiter (\\t)")) -> ()  [unwired: 9 in, 2 out]
      }
    }
    n138 = Multiply(x=1000000.0, y=w56) -> (x*y=w150:fxp<+/-,64,32>[])
    n139 = case shown="False" "RF Power normalize" {
      tunnel: w109 -> [w176 w179]
      tunnel: [w176 w178] -> w58
      tunnel: w57 -> [_ w177]
      frame False {
      }
      frame True {
        n140 = Multiply(x=w179, y=w177) -> (x*y=w178:dbl[])
      }
    }
    n141 = Or Array Elements(Boolean array=w40) -> (logical OR=w39:bool)
    n142 = Divide(x=w141, y=100.0) -> (x/y=w54:dbl[])
    n143 = call "Power normalization.vi"("% of max CH 1"="% of max CH 1", "CH 1 frequency"=w56, "% of max CH 0"="% of max CH 0", "CH 0 frequency"=w59) -> ("Normalized CH1"=w104:dbl[], "Normalized CH 0"=w106:dbl[])
    n144 = Divide(x=w152, y=fxp<+,32,16> 6103.515625) -> (x/y=w115:fxp<+,30,14>[])
    n145 = Divide(x=w150, y=fxp<+,32,16> 6103.515625) -> (x/y=w114:fxp<+,30,14>[])
    n146 = Multiply(x=w58, y=w106) -> (x*y=w110:fxp<+,32,5>[])
    n147 = case shown="True" "RF Power normalize" {
      tunnel: [w172 w175] -> w55
      tunnel: w54 -> [w172 w174]
      tunnel: w53 -> [_ w173]
      frame False {
      }
      frame True {
        n148 = Multiply(x=w173, y=w174) -> (x*y=w175:dbl[])
      }
    }
    n149 = Multiply(x=w104, y=w55) -> (x*y=w105:fxp<+,32,5>[])
    n150 = case shown="True" w39 {
      tunnel: w163 -> [w181 w189]
      tunnel: w162 -> [w180 w188]
      tunnel: [w181 w187] -> w160
      tunnel: [w180 w186] -> w159
      tunnel: w115 -> [_ w185]
      tunnel: w114 -> [_ w184]
      tunnel: w110 -> [_ w183]
      tunnel: w105 -> [_ w182]
      frame False {
      }
      frame True {
        n151 = xnode "Read/Write Control"("FPGA VI Reference In"=w189, "error in"=w188, "Wave 1"=w185, "Amp 1"=w183, "Wave 2"=w184, "Amp 2"=w182) -> ("FPGA VI Reference Out"=w187:refnum<k20>, "error out"=w186:errorcluster)
      }
    }
    n152 = In Range and Coerce(upper limit=u8 150, x="# of beams", lower limit=u8 1) -> (coerced(x)=w35:u8)  [unwired: 1 out]
    n153 = local write "# of beams"(w35) -> ()
    n154 = Multiply(x=100, y="Time per beam in us") -> (x*y=w71:i32)
    n155 = Multiply(x=100, y="Signal Delay (us)") -> (x*y=w68:i32)
    n156 = Subtract(x=w71, y="Remove transition edges") -> (x-y=w69:i32)
    n157 = Subtract(x=w69, y=w68) -> (x-y=w67:i32)
    n158 = xnode "Read/Write Control"("FPGA VI Reference In"=w160, "error in"=w159, "Size"=w35, "Timeshare"=w71, "Edge size"="Remove transition edges", "Pass selector"="Input pass through\nmode", "Gains X"="Gains X", "setpoint weighting"="setpoint weighting", "output range"="output range", "X reset? (F)"="X reset? (F)", "Signal Delay"=w68, "Data collection size"=w67) -> ("FPGA VI Reference Out"=w92:refnum<k20>, "error out"=w93:errorcluster)
    n159 = xnode "Read/Write Control"("FPGA VI Reference In"=w92, "error in"=w93, "Apply feedback"="Apply feedback", "Feedback scaling y"="Feedback scaling y", "Feedback scaling x"="Feedback scaling x", "Feedback scaling z"="Feedback scaling z", "Gains Y"="Gains Y", "setpoint weighting 2"="setpoint weighting 2", "output range 2"="output range 2", "Y reset? (F)"="Y reset? (F)", "Gains Z"="Gains Z", "setpoint weighting 3"="setpoint weighting 3", "output range 3"="output range 3", "Z reset? (F)"="Z reset? (F)", "Set Point Initialization"="Set Point Initialization") -> ("FPGA VI Reference Out"=w91:refnum<k20>, "error out"=w89:errorcluster, "actions 2"=→"actions 2":T8, "output 2"=→"output 2":sgl, "error 2"=→"error 2":sgl, "actions 3"=→"actions 3":T8, "output 3"=→"output 3":sgl, "error 3"=→"error 3":sgl, "actions"=→"actions":T8, "output"=→"output":sgl, "error"=→"error":sgl)
    n160 = Or(x="stop", y=w89) -> (x .or. y?=w95:bool)
    n161 = in-place {
      in-place-border: [w315] -> w96
      in-place-border: w95 -> [w313]
      n162 = in-place-dvr #10(w166) -> (w316:bool, w314:errorcluster)
      n163 = Compound Arithmetic op=OR(w313, w316, w314) -> (w315:bool)
      n164 = in-place-dvr #10(w315) -> ()  [unwired: 2 out]
    }
    n165 = Wait (ms)(milliseconds to wait=u32 33) -> ()  [unwired: 1 out]
  }
  n166 = while {
    tunnel: [w411] -> _
    tunnel: w3 -> [w410]
    tunnel: w13 -> [w394]
    tunnel: w1 -> [w407]
    tunnel: w6 -> [w409]
    tunnel: [w398] -> w10
    tunnel: w12 -> [w384]
    stop <- w408 stop-if-true
    w388 = 0  # Waveform recording stream index
    # "The example interleaves 4 channels of data into one stream."
    # "Wait for the transfer to complete.  This will report overflows if they occur during the transfer."
    # "Configure the AI stream for a finite recording and start"
    # "Configure the input channel and trigger"
    # "Analog Input"
    n167 = local read "# of beams"() -> (w359:u8)
    n168 = call "Volts to Codes.vi"("range (Vpp)"=w394, "Number of Bits"=i16 16, "Volts In"="Data Trigger Level (V)") -> ("ADC Codes Out"=w395:i16)  [unwired: 8 in]
    n169 = case shown="True" "Data transfer method" {
      tunnel: "Record Size" -> [w422 w425]
      tunnel: [w422 w423] -> w373
      tunnel: w359 -> [_ w426]
      frame False {
      }
      frame True {
        n170 = Quotient & Remainder(x=w425, y=w426) -> (x-y*floor(x/y)=w424:u32)  [unwired: 1 out]
        n171 = Subtract(x=w425, y=w424) -> (x-y=w423:u32)
        n172 = local write "Record Size"(w423) -> ()
      }
    }
    n173 = Bundle By Name(cluster=T9 {"level"=0, "trigger when"=enum."Trigger Above"} ("Trigger Configuration"), "level"=w395, "trigger when"="Data Trigger When") -> (w387:T9)
    n174 = xnode "Read/Write Control"("FPGA VI Reference In"=w410, "error in"=w409, "Trigger Type"="Trigger Type", "Trigger Configuration"=w387, "Data transfer method"="Data transfer method", "Downsample"="Downsample") -> ("FPGA VI Reference Out"=w392:refnum<k20>, "error out"=w391:errorcluster)
    n175 = feedback-in #11("Data transfer method") -> ()
    n176 = feedback #11() -> (w374:bool)  [unwired: 1 in]
    n177 = Not Equal?(x=w374, y="Data transfer method") -> (x != y?=w375:bool)
    n178 = case shown="True" w375 {
      tunnel: w373 -> [w427 _]
      tunnel: [w427 w430] -> w372
      tunnel: w359 -> [_ w428]
      frame False {
      }
      frame True {
        n179 = Multiply(x=w428, y=100) -> (x*y=w430:u32)
        n180 = local write "Record Size"(w430) -> ()
      }
    }
    n181 = call <instrlib>:"Clear Stream.vi"("error in (no error)"=w391, "stream index"=w388, "refnum in"=w392) -> ("error out"=w390:errorcluster, "refnum out"=w389:refnum<k20>)  [unwired: 7 in]
    n182 = Multiply(x=u16 4 ("y"), y=w372) -> (x*y=w393:u32)
    n183 = call-poly <instrlib>:"Start Stream.vi"("error in (no error)"=w390, "num samples"=w393, "stream index"=w388, "refnum in"=w389) -> ("error out"=w403:errorcluster, "refnum out"=w401:refnum<k20>)  [unwired: 6 in]
    n184 = local read "Time per beam in us"() -> (w380:i32)
    n185 = call-poly <instrlib>:"Wait.vi"("error in (no error)"=w403, "stream index"=w388, "refnum in"=w401) -> ("error out"=w399:errorcluster, "samples transferred"=w402:u64, "refnum out"=w400:refnum<k20>)  [unwired: 5 in, 1 out]
    n186 = Multiply(x=100, y=w380) -> (x*y=w370:i32)
    n187 = case shown="True" "Data transfer method" {
      tunnel: w384 -> [w439 w442]
      tunnel: [w438 w440] -> w383
      tunnel: "Downsample" -> [w437 _]
      tunnel: w370 -> [_ w441]
      frame False {
        n188 = Divide(x=w439, y=w437) -> (x/y=w438:dbl)
      }
      frame True {
        n189 = Divide(x=w442, y=w441) -> (x/y=w440:dbl)
      }
    }
    n190 = xnode "Invoke Method"("FPGA VI Reference In"=w400, "error in"=w399, "Number of Elements"=w402) -> ("FPGA VI Reference Out"=w411:refnum<k20>, "error out"=w398:errorcluster, "Data"=w379:i16[])  [unwired: 1 in, 1 out]
    n191 = call "Scale Acquired Data + Separate Timeshare Data.vi"("Data In"=w379, "Number of Bits"=i16 16, "Sample Rate"=w383, "Array size"=w359, "range (V)"=w394, "Timeshare sampling"="Data transfer method") -> ("Beam sorted X data"=w366:dbl[][], "AI stream sampling rate"=w361:dbl, "Beam sorted Y data"=w365:dbl[][], "Beam sorted sampling rate"=w362:dbl, "Beam sorted SUM data"=w364:dbl[][], "Data"=→"AI":waveform(dbl)[], "X Data"=w378:waveform(dbl)[], "AI stream data"=w363:dbl[][], "Y Data"=w377:waveform(dbl)[], "SUM Data"=w376:waveform(dbl)[])  [unwired: 4 in]
    n192 = case shown="True" "Data transfer method" {
      tunnel: w378 -> [_ w436]
      tunnel: w377 -> [_ w432]
      tunnel: w376 -> [_ w431]
      frame False {
      }
      frame True {
        n193 = call-poly <vilib>:"FFT Power Spectrum and PSD.vi"("time signals"=w436) -> ("Power Spectrum / PSD"=→"X PSD":cluster{"f0":dbl, "df":dbl, "magnitude":dbl[]}[])  [unwired: 7 in, 3 out]
        n194 = call-poly <vilib>:"FFT Power Spectrum and PSD.vi"("time signals"=w432) -> ("Power Spectrum / PSD"=→"Y PSD":cluster{"f0":dbl, "df":dbl, "magnitude":dbl[]}[])  [unwired: 7 in, 3 out]
        n195 = call-poly <vilib>:"FFT Power Spectrum and PSD.vi"("time signals"=w431) -> ("Power Spectrum / PSD"=→"SUM PSD":cluster{"f0":dbl, "df":dbl, "magnitude":dbl[]}[])  [unwired: 7 in, 3 out]
        "X" <- w436
        "Y" <- w432
        "SUM" <- w431
      }
    }
    n196 = call "check_folder.vi"("path in"="Save Path Directory") -> ("path out"=w368:path)
    n197 = case shown="True" "Save data" {
      tunnel: w368 -> [_ w421]
      tunnel: "File name" -> [_ w420]
      tunnel: w366 -> [_ w419]
      tunnel: w365 -> [_ w418]
      tunnel: w364 -> [_ w417]
      tunnel: w363 -> [_ w416]
      tunnel: w362 -> [_ w415]
      tunnel: w361 -> [_ w414]
      tunnel: "Data transfer method" -> [_ w413]
      frame False {
      }
      frame True {
        n198 = call "save_data.vi"("AI stream data"=w416, "Beam sorted SUM data"=w417, "Beam sorted Y data"=w418, "Beam sorted X data"=w419, "Collection type"=w413, "File name"=w420, "Save Path Directory"=w421, "AI stream sampling rate"=w414, "Beam sorted sampling rate"=w415) -> ()
      }
    }
    n199 = in-place {
      in-place-border: [w444] -> w408
      in-place-border: w398 -> [w446]
      n200 = in-place-dvr #12(w407) -> (w445:bool, w443:errorcluster)
      n201 = Compound Arithmetic op=OR(w446, w445, w443) -> (w444:bool)
      n202 = in-place-dvr #12(w444) -> ()  [unwired: 2 out]
    }
    n203 = Wait (ms)(milliseconds to wait=u32 100) -> ()  [unwired: 1 out]
  }
  n204 = Merge Errors(w10, w9) -> (w11:errorcluster)
  n205 = xnode "Read/Write Control"("FPGA VI Reference In"=w17, "error in"=w11, "stream.request state 2"=3) -> ("FPGA VI Reference Out"=w14:refnum<k20>, "error out"=w16:errorcluster)
  n206 = xnode "Close FPGA VI Reference"("FPGA VI Reference In"=w14, "error in"=w16) -> ("error out"=w24:errorcluster)
  n207 = call <vilib>:"Simple Error Handler.vi"("error in (no error)"=w24) -> ("error out"=→"Error Out":errorcluster)  [unwired: 4 in, 4 out]
